vi "uActor_Launch__Synchronous.vi"(6 "Show FP (F)":bool, 8 "error in (no error)":errorcluster, 10 "Actor to Launch":refnum<class "uActor.lvclass">, 11 "Caller Actor in":refnum<class "uActor.lvclass">) -> (0 "error out":errorcluster, 2 "uTransport_uActor":refnum<class "uTransport_uActor.lvclass">, 3 "Caller Actor out":refnum<class "uActor.lvclass">)   [LabVIEW 2023, in "uFramework.lvlib" / "uActor.lvclass"]
doc: "Launch a new Actor and block dataflow until verifying that the actor has initialized internally and is ready to reach to incoming messages. \n\nThis will be a root actor if no caller actors are wired in."
uses:
  uActor.lvclass
  uActor.lvclass/uActor.ctl
  uTransport_uActor/uTransport_uActor.lvclass
panel:
  in  "timeout in ms (5000)":i32=1000
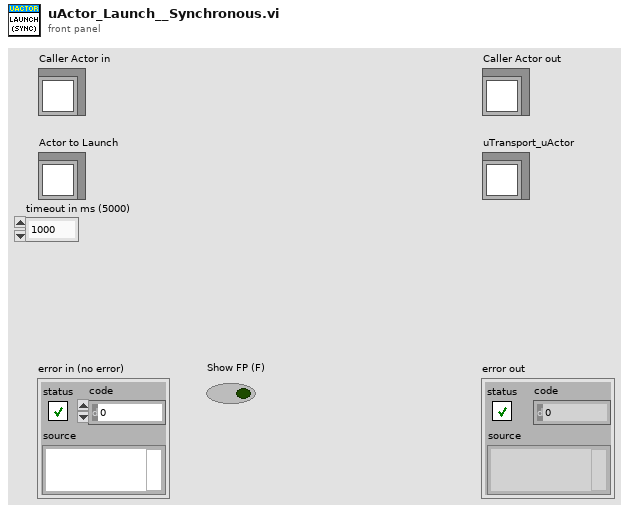
[diagram p1: front panel]
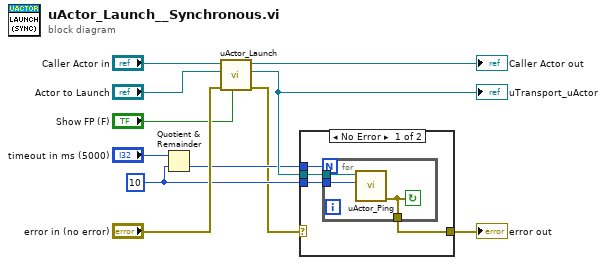
[diagram p0: block diagram]
diagram:
  w3 = 10 ("timeout in ms (1000)")
  n1 = Quotient & Remainder(x="timeout in ms (5000)", y=w3) -> (floor(x/y)=w4:i32)  [unwired: 1 out]
  n2 = call "uActor_Launch.vi"("Show FP (F)"="Show FP (F)", "error in (no error)"="error in (no error)", "Actor to Launch"="Actor to Launch", "Caller Actor in"="Caller Actor in") -> ("error out"=w2:errorcluster, "uTransport_uActor"=w6:refnum<class "uTransport_uActor.lvclass">, "Caller Actor out"=→"Caller Actor out":refnum<class "uActor.lvclass">)  [unwired: 5 in]
  "uTransport_uActor" <- w6
  n3 = case shown="No Error" w2 {
    selector: w2 -> [_ w19]
    tunnel: w6 -> [w15 _]
    tunnel: w4 -> [w14 _]
    tunnel: w3 -> [w13 _]
    tunnel: [w12 w19] -> w1
    frame No Error {
      n4 = for {
        N: w14 -> [_]
        tunnel: w15 -> [w18]
        tunnel: [w16] -> w12
        tunnel: w13 -> [w17]
        stop <- w16 continue-if-true
        n5 = call "uActor_Ping.vi"("timeout in ms (1000)"=w17, "uActor Transport"=w18) -> ("error out"=w16:errorcluster)  [unwired: 8 in, 1 out]
      }
    }
    frame Error {
    }
  }
  "error out" <- w1
